vi "EFW Get Num.vi"(8 "error in (no error)":errorcluster caption="错误输入（无错误）") -> (0 "error out":errorcluster caption="错误输出", 3 "function return":i32)   [LabVIEW 2012, in "EFW_filter.lvlib"]
doc: "EFW_API int EFWGetNum();"
uses:
  <userlib>/EFW_filter/EFW_filter.lvlib
  <userlib>/EFW_filter/EFW_filter.dll
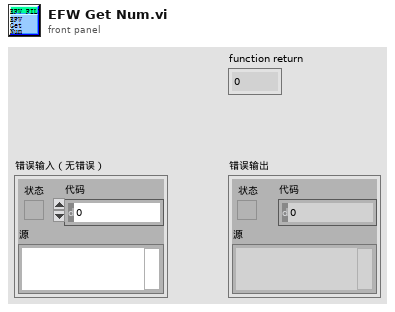
[diagram p1: front panel]
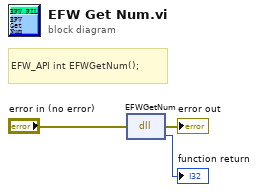
[diagram p0: block diagram]
diagram:
  # "EFW_API int EFWGetNum();"
  n1 = dll-call lib="D:/Program Files (x86)/National Instruments/LabVIEW 2012/user.lib/EFW_filter/EFW_filter.*" fn="EFWGetNum"(error in="error in (no error)") -> (error out=→"error out":errorcluster, →"function return":i32)  [unwired: 2 in, 1 out]
